vi "Change Icon Template.vi"(8 "error in (no error)":errorcluster, 9 "Template Path":path, 11 "vi reference":refnum<vi>) -> (0 "error out":errorcluster, 3 "reference out":refnum<vi>)   [LabVIEW 2015]
panel:
  in  "Path":path
  in  "Icon":picture
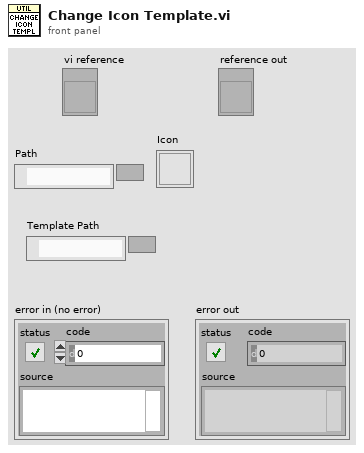
[diagram p1: front panel]
types:
  T1 = typedef "imagedata.ctl" = cluster{"image type":i32, "image depth":i32, "image":u8[], "mask":u8[], "colors":u32[], "Rectangle":cluster{"left":i16, "top":i16, "right":i16, "bottom":i16}}
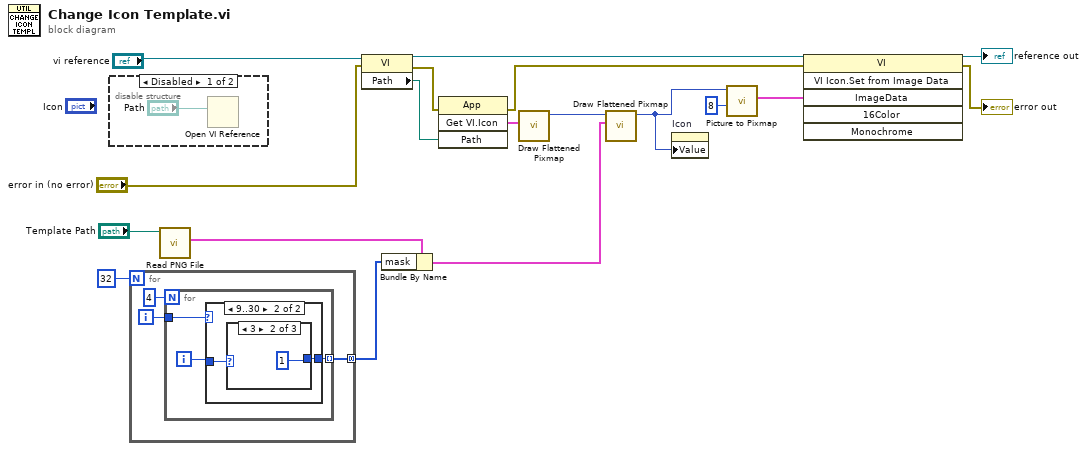
[diagram p0: block diagram]
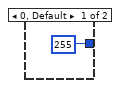
[diagram p3: hidden frame]
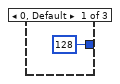
[diagram p4: hidden frame]
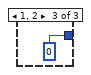
[diagram p5: hidden frame]
diagram:
  n1 = disable-structure shown="Disabled" {
    frame Disabled {
      n2 = Open VI Reference(vi path="Path") -> ()  [unwired: 5 in, 2 out]
    }
    frame Enabled {
    }
  }
  n3 = for {
    N: 32 -> [_]
    tunnel: [w21] -> w3 mode=concatenating
    i -> [w22]
    n4 = for {
      N: 4 -> [_]
      tunnel: w22 -> [w24]
      tunnel: [w25] -> w21 mode=indexing
      i -> [w23]
      n5 = case shown="9..30" w24 {
        tunnel: [u8 255 w27] -> w25
        tunnel: w23 -> [_ w28]
        frame 0, Default {
        }
        frame 9..30 {
          n6 = case shown="3" w28 {
            tunnel: [u8 128 u8 1 u8 0] -> w27
            frame 0, Default {
            }
            frame 3 {
            }
            frame 1, 2 {
            }
          }
        }
      }
    }
  }
  n7 = call <vilib>:"Read PNG File.vi"("path to PNG file"="Template Path") -> ("image data"=w7:T1)  [unwired: 8 in, 2 out]
  n8 = property class="VI"(reference="vi reference", error in="error in (no error)") -> (reference out=w11:refnum<vi>, error out=w9:errorcluster, "Path"=w10:path)
  n9 = Bundle By Name(cluster=w7, "mask"=w3) -> (w4:T1)
  n10 = invoke class="App" method="Get VI.Icon"(error in=w9, "Path"=w10) -> (error out=w14:errorcluster, "Get VI.Icon"=w18:T1)  [unwired: 2 in, 2 out]
  n11 = call <vilib>:"Draw Flattened Pixmap.vi"("image data"=w18) -> ("new picture"=w6:picture)  [unwired: 8 in]
  n12 = call <vilib>:"Draw Flattened Pixmap.vi"("image data"=w4, "picture"=w6) -> ("new picture"=w5:picture)  [unwired: 7 in]
  n13 = property on="Icon" class="Pict"("Value"=w5) -> ()  [unwired: 2 in, 2 out]
  n14 = call <vilib>:"Picture to Pixmap.vi"("depth"=8, "picture"=w5) -> ("image data"=w15:T1)  [unwired: 8 in, 1 out]
  n15 = invoke class="VI" method="VI Icon.Set from Image Data"(reference=w11, error in=w14, "ImageData"=w15) -> (reference out=→"reference out":refnum<vi>, error out=→"error out":errorcluster)  [unwired: 3 in, 4 out]
